vi "MD5, Is Match.vi"(0 "MD5(b)":string, 1 "MD5(a)":string) -> (2 "matches":bool[](array[boolean]), 3 "MD5 match":bool, 4 "sizeof MD5(b)":i32, 5 "MD5(b)":string[](array[string]), 6 "sizeof MD5(a)":i32, 7 "MD5(a)":string[](array[string]))   [LabVIEW 2010]
doc: "This function performs a character by character comparison of two MD5 message-digest strings.\n\nThe \"MD5 Match\" indicator will be TRUE when both MD5 message-digests contain 32 characters and all characters match."
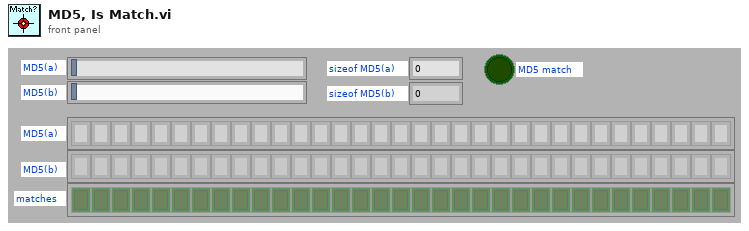
[diagram p1: front panel]
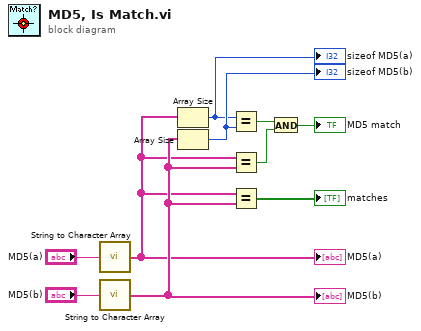
[diagram p0: block diagram]
diagram:
  n1 = call "String to Character Array.vi"("input string"="MD5(a)") -> ("character array"=w3:string[])
  "MD5(a)" <- w3
  n2 = call "String to Character Array.vi"("input string"="MD5(b)") -> ("character array"=w4:string[])
  "MD5(b)" <- w4
  n3 = Array Size(array=w3) -> (size(s)=w1:i32)
  "sizeof MD5(a)" <- w1
  n4 = Array Size(array=w4) -> (size(s)=w2:i32)
  "sizeof MD5(b)" <- w2
  n5 = Equal?(x=w1, y=w2) -> (x = y?=w7:bool)
  n6 = Equal?(x=w3, y=w4) -> (x = y?=w6:bool)
  n7 = Equal?(x=w3, y=w4) -> (x = y?=→"matches":bool[])
  n8 = And(x=w7, y=w6) -> (x .and. y?=→"MD5 match":bool)
